vi "读取-写入新值清空.vi"(8 "error in (no error)":errorcluster caption="错误输入（无错误）", 11 "计算器类 输入":refnum<class "计算器类.lvclass">) -> (0 "error out":errorcluster caption="错误输出", 3 "计算器类 输出":refnum<class "计算器类.lvclass">)   [LabVIEW 2020, in "计算器类.lvclass"]
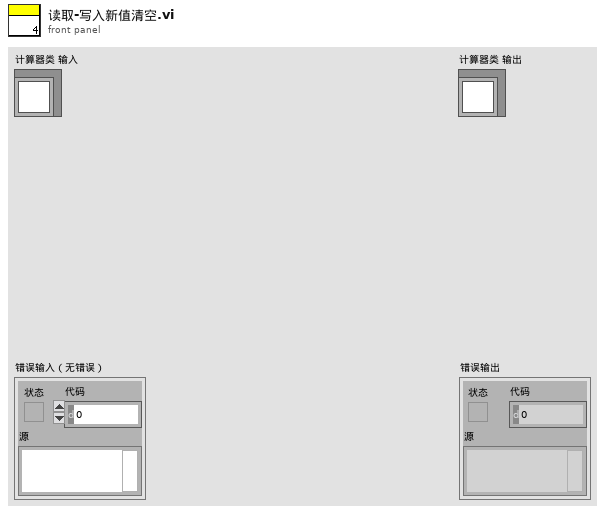
[diagram p1: front panel]
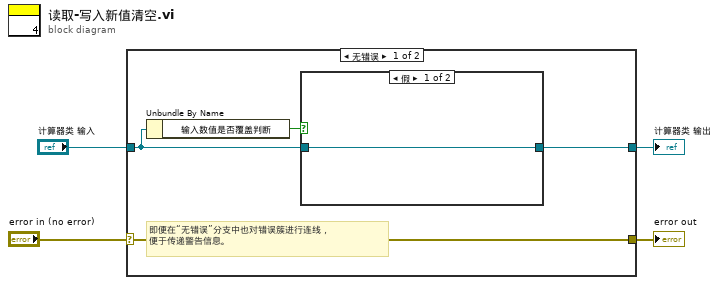
[diagram p0: block diagram]
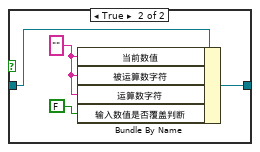
[diagram p2: hidden frame]
diagram:
  n1 = case shown="无错误" "error in (no error)" {
    selector: "error in (no error)" -> [w8 w15]
    tunnel: [w8 w15] -> w3
    tunnel: [w6 w14] -> w1
    tunnel: "计算器类 输入" -> [w5 w14]
    frame No Error {
      # "即便在“无错误”分支中也对错误簇进行连线，\n便于传递警告信息。"
      n2 = Unbundle By Name(w5) -> ("输入数值是否覆盖判断"=w7:bool)
      n3 = case shown="假" w7 {
        tunnel: [w9 w11] -> w6
        tunnel: w5 -> [w9 w10]
        frame False {
        }
        frame True {
          w12 = "" ("赋值变量")
          n4 = Bundle By Name(cluster=w10, "当前数值"=w12, "被运算数字符"=w12, "运算数字符"=w12, "输入数值是否覆盖判断"=FALSE) -> (w11:refnum<class "计算器类.lvclass">)
        }
      }
    }
    frame Error {
    }
  }
  "error out" <- w3
  "计算器类 输出" <- w1
